vi "Test - Thermal Chamber Controller_DQMH - Update Set Point 1-teardown.vi"(7 "test case ID":string, 8 "error in (no error)":errorcluster, 10 "Temperature Set Point":dbl format="%#_13g", 11 "no error":bool) -> (0 "error out":errorcluster, 3 "result":bool)   [LabVIEW 2015]
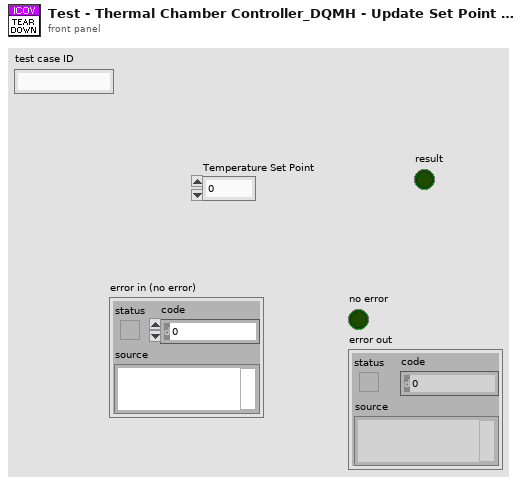
[diagram p1: front panel]
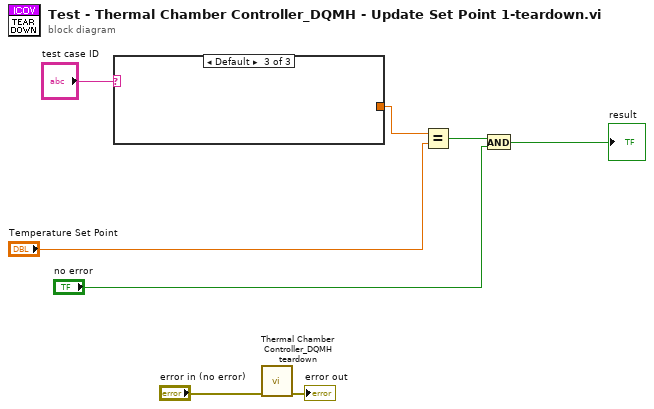
[diagram p0: block diagram]
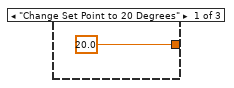
[diagram p2: hidden frame]
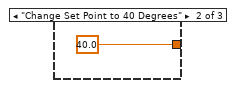
[diagram p3: hidden frame]
diagram:
  n1 = case shown="Default" "test case ID" {
    tunnel: [20.0 ("Temperature Set Point 2") 40.0 ("Temperature Set Point 2") _] -> w1
    frame "Change Set Point to 20 Degrees" {
    }
    frame "Change Set Point to 40 Degrees" {
    }
    frame Default {
    }
  }
  n2 = call "Thermal Chamber Controller_DQMH teardown.vi"("error in (no error)"="error in (no error)") -> ("error out"=→"error out":errorcluster)  [unwired: 10 in]
  n3 = Equal?(x=w1, y="Temperature Set Point") -> (x = y?=w7:bool)
  n4 = And(x=w7, y="no error") -> (x .and. y?=→"result":bool)
